vi "Read channels.vi"(8 "error in (no error)":errorcluster, 11 "Wait On Integer Config in":refnum<class "Wait On Integer Config.lvclass">) -> (0 "error out":errorcluster, 2 "Channels":refnum<class "TBM channel.lvclass">[](array[class]), 3 "Wait On Integer Config out":refnum<class "Wait On Integer Config.lvclass">)   [LabVIEW 2018, in "Wait On Integer Config.lvclass"]
uses:
  Wait On Integer Config.lvclass
  <vilib>/NI/Tag Bus Module Framework/channel/TBM channel.lvclass
  Wait On Integer Config.lvclass/Wait On Integer Config.ctl
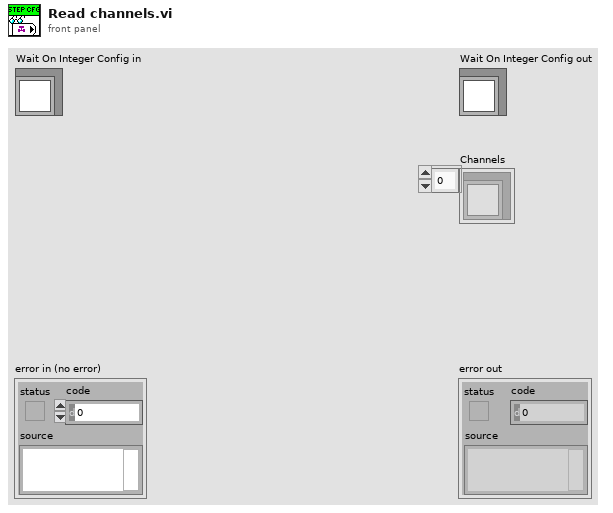
[diagram p1: front panel]
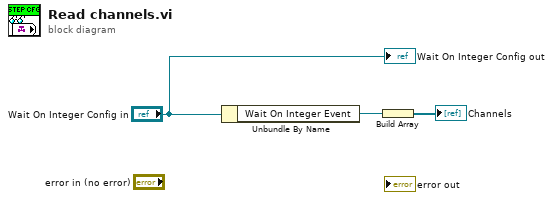
[diagram p0: block diagram]
diagram:
  n1 = Unbundle By Name("Wait On Integer Config in") -> ("Wait On Integer Event"=w3:refnum<class "TBM channel.lvclass">)
  n2 = Build Array(w3) -> (→"Channels":refnum<class "TBM channel.lvclass">[])
  "Wait On Integer Config out" <- "Wait On Integer Config in"
